vi "Test Case, Master Record Results.vi"() -> ()   [LabVIEW 2010]
uses:
  MyCalc/Active Output Test Cases.ctl
  MyCalc/Analyze Ouptut Parameters.ctl
  Generic/Waveform Attribute/Waveform Attribute Cluster.ctl
panel:
  in  "error in":errorcluster
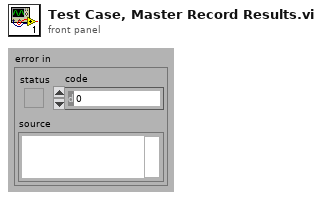
[diagram p1: front panel]
types:
  T1 = typedef "Waveform Attribute Cluster.ctl" = cluster{"Label":string, "Value":dbl}
  T2 = typedef "Analyze Ouptut Parameters.ctl" = cluster{"Stim Amplitude":dbl[], "Stim Pulse Width":dbl[], "Interphase Delay":dbl[], "Recovery Amplitude":dbl[], "Recovery PW":dbl[], "Recovery Holdoff":dbl[], "Frequency":dbl, "Avg CBC Width":dbl, "Avg. CBC Holdoff":dbl, "Avg. CBC Amplitude":dbl}
  T3 = typedef "Active Output Test Cases.ctl" = string
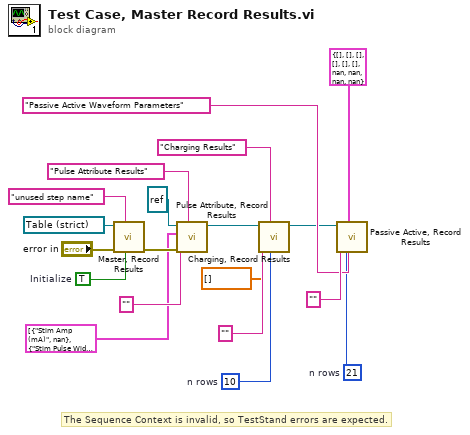
[diagram p0: block diagram]
diagram:
  w4 = 21  # n rows
  w5 = 10  # n rows
  w18 = TRUE  # Initialize
  # "The Sequence Context is invalid, so TestStand errors are expected."
  n1 = call "Master, Record Results.vi"("Initialize (F)"=w18, "step name"="unused step name", "error in"="error in", "Tbl Refnum"=refnum<vi> refnum) -> ("error out"=w15:errorcluster)  [unwired: 6 in, 1 out]
  n2 = call "Pulse Attribute, Record Results.vi"("step name"="Pulse Attribute Results", "error in"=w15, "test case"=T3 "", "results"=T1[] [{"Label"="Stim Amp (mA)", "Value"=nan}, {"Label"="Stim Pulse Width (us)", "Value"=nan}, {"Label"="Interphase Delay (us)", "Value"=nan}, {"Label"="Recvy Amp (mA)", "Value"=nan}, {"Label"="Recvy Pulse Width (us)", "Value"=nan}, {"Label"="Frequency (Hz)", "Value"=nan}, {"Label"="Period Jitter (us rms)", "Value"=nan}], "Sequence Context"=refnum<k7> refnum) -> ("Sequence Context dup"=w2:refnum<k7>)  [unwired: 5 in, 1 out]
  n3 = call "Charging, Record Results.vi"("n rows"=w5, "step name"="Charging Results", "test case"=T3 "", "Numeric Results"=dbl[] [], "Sequence Context"=w2) -> ("Sequence Context dup"=w1:refnum<k7>)  [unwired: 5 in, 1 out]
  n4 = call "Passive Active, Record Results.vi"("step name"="Passive Active Waveform Parameters", "Waveform Parameters"=T2 {"Stim Amplitude"=[], "Stim Pulse Width"=[], "Interphase Delay"=[], "Recovery Amplitude"=[], "Recovery PW"=[], "Recovery Holdoff"=[], "Frequency"=nan, "Avg CBC Width"=nan, "Avg. CBC Holdoff"=nan, "Avg. CBC Amplitude"=nan}, "n rows"=w4, "test case"=T3 "", "Sequence Context"=w1) -> ()  [unwired: 5 in, 2 out]
